vi "Get Report Settings.vi"(0 "report in":refnum<class "NI_Standard Report.lvclass">, 11 "error in (no error)":errorcluster) -> (4 "report out":refnum<class "NI_Standard Report.lvclass">, 6 "text options":T1, 10 "font settings":T2, 14 "text color":u32(colorbox), 15 "error out":errorcluster)   [LabVIEW 2017, in "NI_Standard Report.lvclass"]
doc: "Retrieves information about the current font and text settings of a given report."
uses:
  <vilib>/Utility/NIReport.llb/Standard Report/NI_Standard Report.lvclass
  <vilib>/Utility/NIReport.llb/Standard Report/NI_Standard Report.lvclass/NI_Standard Report.ctl
  <vilib>/Utility/NIReport.llb/NI_ReportGenerationCore.lvlib
panel:
  out "color - RGB":cluster{"red":u8, "green":u8, "blue":u8}
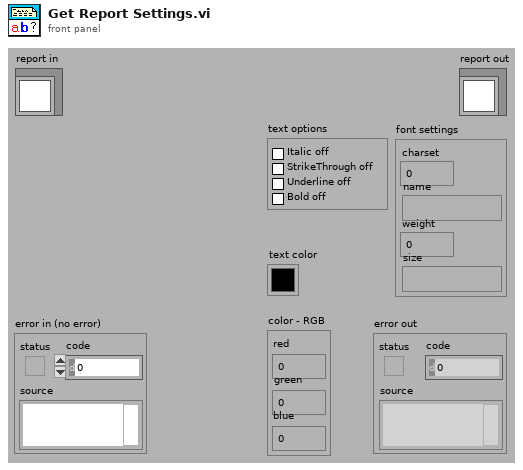
[diagram p1: front panel]
types:
  T1 = cluster{"Italic":bool, "StrikeThrough":bool, "Underline":bool, "Bold":bool}
  T2 = cluster{"charset":i16, "name":string, "weight":i16, "size":string}
  T3 = cluster{"Italic":bool, "Strikethrough":bool, "Underline":bool, "Bold":bool}
  T4 = cluster{"Charset":i16, "Name":string, "Weight":i16, "Size":string}
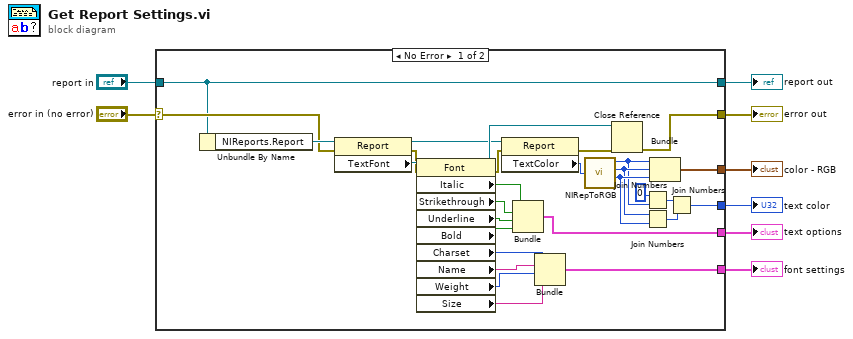
[diagram p0: block diagram]
diagram:
  n1 = case shown="No Error" "error in (no error)" {
    selector: "error in (no error)" -> [w15 w39]
    tunnel: [w14 w39] -> w7
    tunnel: [w9 w38] -> w5
    tunnel: "report in" -> [w9 w38]
    tunnel: [w13 _] -> w4
    tunnel: [w12 _] -> w3
    tunnel: [w11 _] -> w2
    tunnel: [w10 _] -> w1
    frame No Error {
      n2 = Unbundle By Name(w9) -> ("NIReports.Report"=w16:refnum<k7>)
      n3 = property class="Report"(reference=w16, error in=w15) -> (reference out=w31:refnum<k7>, error out=w22:errorcluster, "TextFont"=w23:refnum<k7>)
      n4 = property class="Font"(reference=w23, error in=w22) -> (reference out=w35:refnum<k7>, error out=w24:errorcluster, "Italic"=w33:bool, "Strikethrough"=w17:bool, "Underline"=w18:bool, "Bold"=w19:bool, "Charset"=w20:i16, "Name"=w36:string, "Weight"=w37:i16, "Size"=w21:string)
      n5 = property class="Report"(reference=w31, error in=w24) -> (error out=w34:errorcluster, "TextColor"=w32:u32)  [unwired: 1 out]
      n6 = Bundle("Italic"=w33, "Strikethrough"=w17, "Underline"=w18, "Bold"=w19) -> (w10:T3)  [unwired: 1 out]
      n7 = Bundle("Charset"=w20, "Name"=w36, "Weight"=w37, "Size"=w21) -> (w13:T4)  [unwired: 1 out]
      n8 = call <vilib>:"NIRepToRGB.vi"("color"=w32) -> ("red"=w25:u8, "green"=w26:u8, "blue"=w27:u8)  [unwired: 1 out]
      n9 = Close Reference(reference=w35, error in (no error)=w34) -> (error out=w14:errorcluster)
      n10 = Join Numbers(hi=u8 0, lo=w25) -> ((hi.lo)=w29:u16)
      n11 = Join Numbers(hi=w26, lo=w27) -> ((hi.lo)=w30:u16)
      n12 = Bundle("red"=w25, "green"=w26, "blue"=w27) -> (w12:cluster{"red":u8, "green":u8, "blue":u8})  [unwired: 1 out]
      n13 = Join Numbers(hi=w29, lo=w30) -> ((hi.lo)=w11:u32)
    }
    frame Error {
    }
  }
  "error out" <- w7
  "report out" <- w5
  "color - RGB" <- w3
  "text color" <- w2
  "text options" <- w1
  "font settings" <- w4
